vi "난수 발생.vi"(10 "대기 시간(ms)":u32=100) -> (2 "웨이브폼 차트":dbl(graph))   [LabVIEW 2014]
panel:
  in  "정지":bool
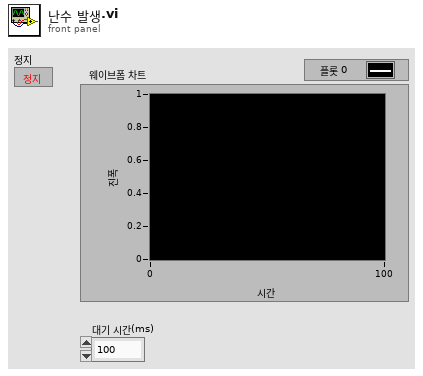
[diagram p1: front panel]
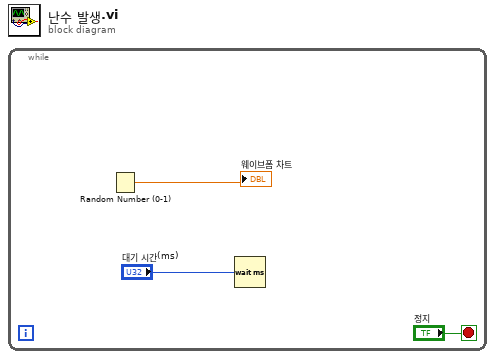
[diagram p0: block diagram]
diagram:
  n1 = while {
    stop <- "정지" stop-if-true
    n2 = Random Number (0-1)() -> (number: 0 to 1=→"웨이브폼 차트":dbl)
    n3 = Wait (ms)(milliseconds to wait="대기 시간(ms)") -> ()  [unwired: 1 out]
  }
